vi "Highlight Execution Logic Error - User Name or Public.vi"() -> ()   [LabVIEW 2015]
panel:
  out "Message":string
  in  "Use Public Profile?":bool
  in  "User Name":string
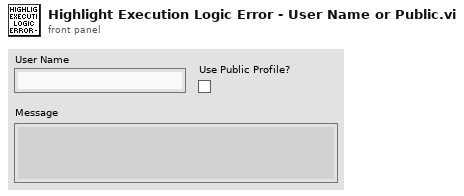
[diagram p1: front panel]
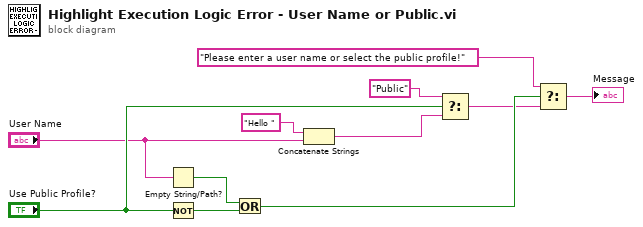
[diagram p0: block diagram]
diagram:
  n1 = Empty String/Path?(string/path="User Name") -> (empty?=w7:bool)
  n2 = Not(x="Use Public Profile?") -> (.not. x?=w6:bool)
  n3 = Or(x=w7, y=w6) -> (x .or. y?=w11:bool)
  n4 = Concatenate Strings "Concatenate Strings"("Hello " ("string"), "User Name") -> (w1:string)
  n5 = Select(t="Public", s="Use Public Profile?", f=w1) -> (s? t:f=w4:string)
  n6 = Select(t="Please enter a user name or select the public profile!" ("f"), s=w11, f=w4) -> (s? t:f=→"Message":string)
